vi "Failsafe.vi"(7 "Name of Experiment":string, 8 "error in":errorcluster, 9 "Emergency Contact (Carrier)":enum16{"T-Mobile", "AT&T", "Verizon", "Sprint"}(ring), 10 "Emergency Contact (phone number)":string, 11 "Process_REF":string) -> (0 "error out":errorcluster)   [LabVIEW 2018]
uses:
  <vilib>/smtpClient/Set Message Text.vi
  <vilib>/smtpClient/LabVIEWSMTPClient.lvlib
panel:
  in  "TLS":bool=TRUE
  in  "Outgoing Mail Server (SMTP)":string="smtp.gmail.com"
  in  "Body":string="Error"
  in  "Password":string="labVIEW123"
  in  "Email":string="krishna16842@gmail.com"
  out "Path Out":path
  in  "Path In":path
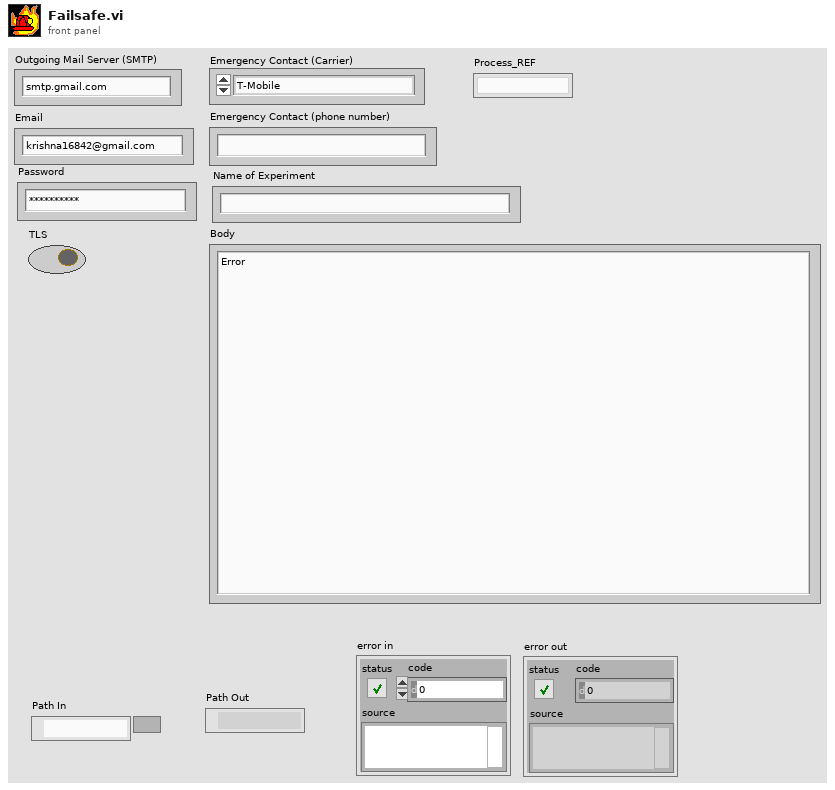
[diagram p1: front panel]
types:
  T1 = typedef "LabVIEWSMTPClient.lvlib/SmtpClientHandle.ctl" = refnum<k1>
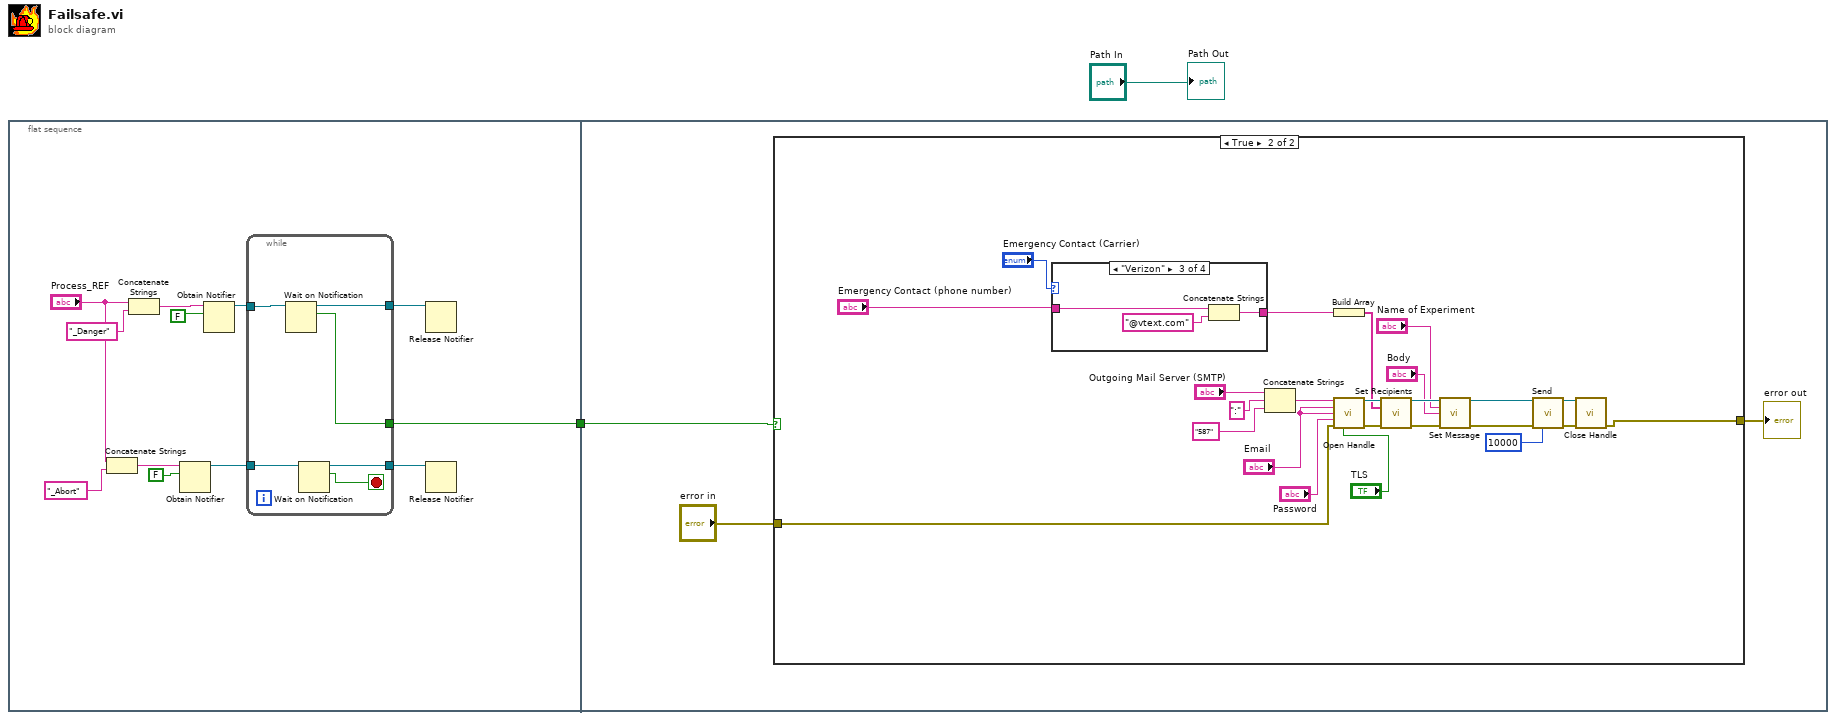
[diagram p0: block diagram]
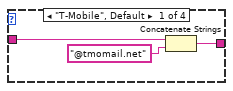
[diagram p3: hidden frame]
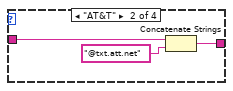
[diagram p4: hidden frame]
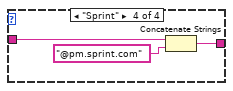
[diagram p5: hidden frame]
diagram:
  n1 = flat-sequence {
    tunnel: [w13] -> w1
    tunnel: w1 -> [w21]
    frame #0 {
      n2 = Concatenate Strings("Process_REF", "_Abort") -> (w6:string)
      n3 = Concatenate Strings("Process_REF", "_Danger") -> (w10:string)
      n4 = Obtain Notifier(name (unnamed)=w6, notification data type=FALSE) -> (notifier out=w7:refnum<notifier>)  [unwired: 2 in, 2 out]
      n5 = Obtain Notifier(name (unnamed)=w10, notification data type=FALSE) -> (notifier out=w8:refnum<notifier>)  [unwired: 2 in, 2 out]
      n6 = while {
        tunnel: w8 -> [w20]
        tunnel: [w19] -> w4
        tunnel: [w18] -> w13
        tunnel: w7 -> [w17]
        tunnel: [w16] -> w3
        stop <- w15 stop-if-true
        n7 = Wait on Notification(notifier=w20) -> (notifier out=w19:refnum<notifier>, notification=w18:bool)  [unwired: 3 in, 2 out]
        n8 = Wait on Notification(notifier=w17) -> (notifier out=w16:refnum<notifier>, notification=w15:bool)  [unwired: 3 in, 2 out]
      }
      n9 = Release Notifier(notifier=w4) -> ()  [unwired: 2 in, 3 out]
      n10 = Release Notifier(notifier=w3) -> ()  [unwired: 2 in, 3 out]
    }
    frame #1 {
      n11 = case shown="True" w21 {
        tunnel: "error in" -> [w24 w26]
        tunnel: [w24 w25] -> w22
        frame False {
        }
        frame True {
          n12 = case shown="\"Verizon\"" "Emergency Contact (Carrier)" {
            tunnel: "Emergency Contact (phone number)" -> [w51 w53 w56 w59]
            tunnel: [w49 w54 w57 w60] -> w34
            frame "T-Mobile", Default {
              n13 = Concatenate Strings(w51, "@tmomail.net" ("string")) -> (w49:string)
            }
            frame "AT&T" {
              n14 = Concatenate Strings(w53, "@txt.att.net" ("string")) -> (w54:string)
            }
            frame "Verizon" {
              n15 = Concatenate Strings(w56, "@vtext.com" ("string")) -> (w57:string)
            }
            frame "Sprint" {
              n16 = Concatenate Strings(w59, "@pm.sprint.com") -> (w60:string)
            }
          }
          n17 = Concatenate Strings("Outgoing Mail Server (SMTP)", ":" ("string"), "587" ("Port")) -> (w29:string)
          n18 = Build Array(w34) -> (w33:string[])
          n19 = call <vilib>:"Open Handle.vi"("server address"=w29, "from"="Email", "username"="Email", "password"="Password", "error in (no error)"=w26, "use TLS (false)"="TLS") -> ("handle out"=w46:T1, "error out"=w43:errorcluster)  [unwired: 8 in]
          n20 = call <vilib>:"Set Recipients.vi"("handle in"=w46, "to"=w33, "error in (no error)"=w43) -> ("handle out"=w42:T1, "error out"=w41:errorcluster)  [unwired: 11 in]
          n21 = call-poly <vilib>:"Set Message.vi"("handle in"=w42, "subject"="Name of Experiment", "plain text message"="Body", "error in (no error)"=w41) -> ("handle out"=w38:T1, "error out"=w37:errorcluster)  [unwired: 10 in]
          n22 = call <vilib>:"Send.vi"("handle in"=w38, "error in (no error)"=w37, "timeout in ms (10000)"=10000) -> ("handle out"=w36:T1, "error out"=w35:errorcluster)  [unwired: 10 in, 1 out]
          n23 = call <vilib>:"Close Handle.vi"("handle in"=w36, "error in (no error)"=w35) -> ("error out"=w25:errorcluster)  [unwired: 12 in, 1 out]
        }
      }
      "error out" <- w22
    }
  }
  "Path Out" <- "Path In"
